vi "Get3DProfile.vi"(9 "dy":dbl, 10 "Origin":cluster{"X":sgl, "Y":sgl, "Z":sgl}, 11 "remaining elements":cluster{"x(mm)":dbl, "y(mm)":dbl, "z(mm)":dbl}[](array[cluster])) -> (0 "Z":dbl[](array[numeric]), 1 "Y":dbl[](array[numeric]), 2 "X":dbl[](array[numeric]), 3 "3D Profile":cluster{"x(mm)":dbl, "y(mm)":dbl, "z(mm)":dbl}[](array[cluster]))   [LabVIEW 2024]
panel:
  out "Z":dbl[](graph)
  out "Y":dbl[](graph)
  out "X":dbl[](graph)
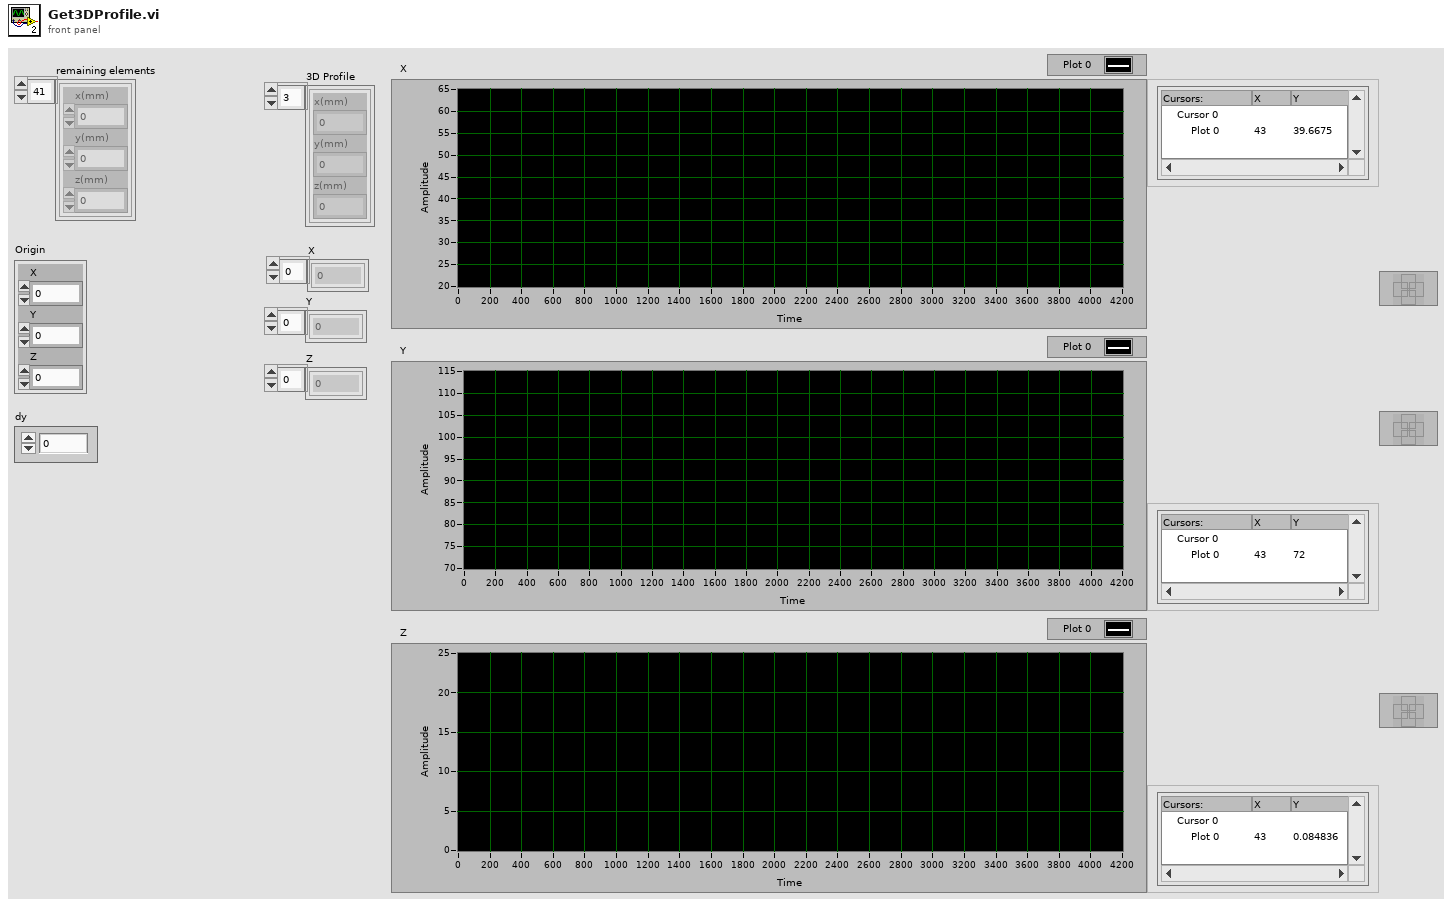
[diagram p1: front panel]
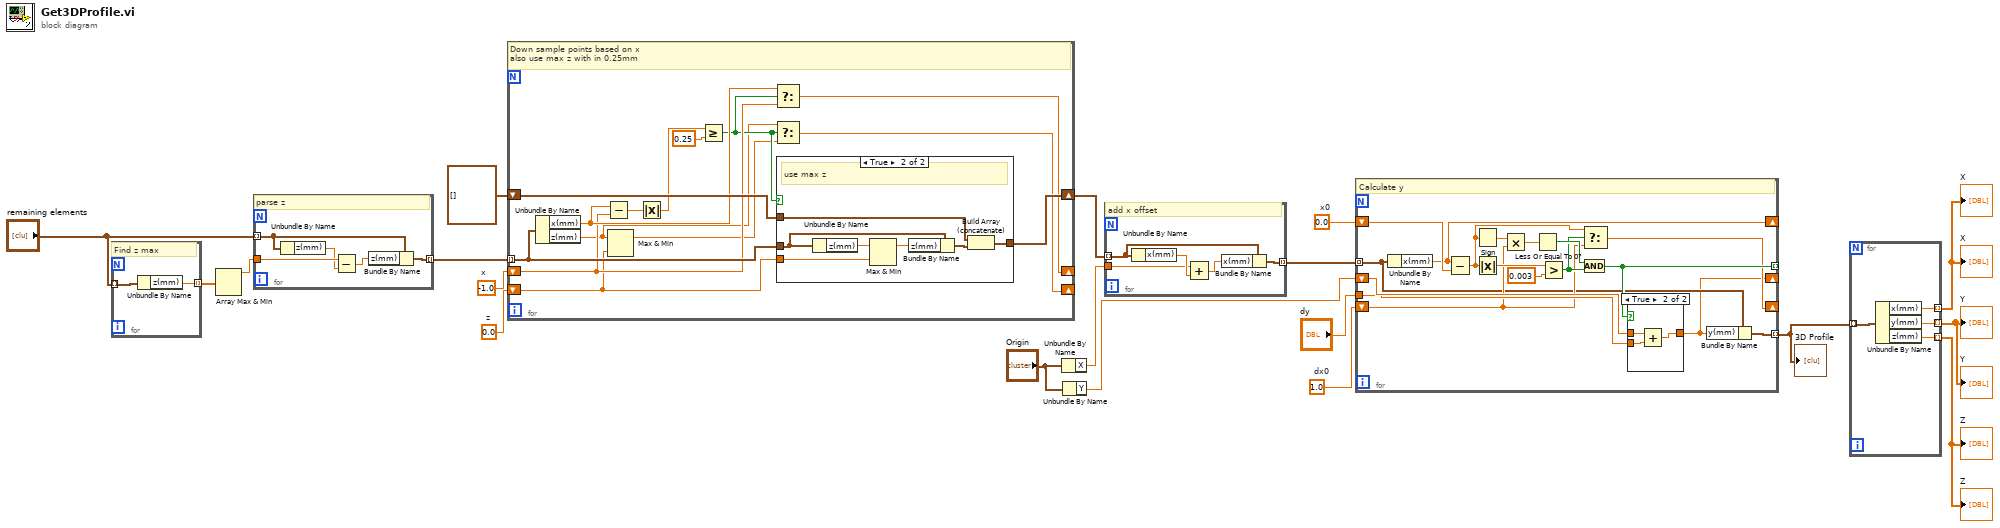
[diagram p0: block diagram]
diagram:
  w6 = 0.0  # z
  w16 = 1.0  # dx0
  w17 = 0.0  # x0
  w18 = -1.0  # x
  n1 = for {
    tunnel: "remaining elements" -> [w21] mode=indexing
    tunnel: [w20] -> w5 mode=indexing
    # "Find z max"
    n2 = Unbundle By Name(w21) -> ("z(mm)"=w20:dbl)
  }
  n3 = Array Max & Min(array=w5) -> (max value=w9:dbl)  [unwired: 3 out]
  n4 = for {
    tunnel: w9 -> [w26]
    tunnel: "remaining elements" -> [w24] mode=indexing
    tunnel: [w22] -> w7 mode=indexing
    # "parse z"
    n5 = Unbundle By Name(w24) -> ("z(mm)"=w25:dbl)
    n6 = Subtract(x=w26, y=w25) -> (x-y=w23:dbl)
    n7 = Bundle By Name(cluster=w24, "z(mm)"=w23) -> (w22:cluster{"x(mm)":dbl, "y(mm)":dbl, "z(mm)":dbl})
  }
  n8 = for {
    tunnel: w7 -> [w37] mode=indexing
    shift-right: [w33] -> _
    shift-left: w18 -> [w34]
    shift-right: [w36] -> w11
    shift-left: cluster{"x(mm)":dbl, "y(mm)":dbl, "z(mm)":dbl}[] [] -> [w38]
    shift-right: [w30] -> _
    shift-left: w6 -> [w27]
    # "Down sample points based on x\nalso use max z with in 0.25mm"
    n9 = Unbundle By Name(w37) -> ("x(mm)"=w35:dbl, "z(mm)"=w29:dbl)
    n10 = Subtract(x=w35, y=w34) -> (x-y=w40:dbl)
    n11 = Max & Min(x=w29, y=w27) -> (max(x,y)=w28:dbl)  [unwired: 1 out]
    n12 = Absolute Value(x=w40) -> (abs(x)=w32:dbl)
    n13 = Greater Or Equal?(x=w32, y=0.25) -> (x >= y?=w31:bool)
    n14 = Select(t=w35, s=w31, f=w34) -> (s? t:f=w33:dbl)
    n15 = Select(t=w29, s=w31, f=w28) -> (s? t:f=w30:dbl)
    n16 = case shown="True" w31 {
      tunnel: w38 -> [w41 w48]
      tunnel: w37 -> [_ w44]
      tunnel: [w41 w47] -> w36
      tunnel: w27 -> [_ w45]
      frame False {
      }
      frame True {
        # "use max z"
        n17 = Unbundle By Name(w44) -> ("z(mm)"=w46:dbl)
        n18 = Max & Min(x=w46, y=w45) -> (max(x,y)=w43:dbl)  [unwired: 1 out]
        n19 = Bundle By Name(cluster=w44, "z(mm)"=w43) -> (w42:cluster{"x(mm)":dbl, "y(mm)":dbl, "z(mm)":dbl})
        n20 = Build Array (concatenate)(w48, w42) -> (w47:cluster{"x(mm)":dbl, "y(mm)":dbl, "z(mm)":dbl}[])
      }
    }
  }
  n21 = Unbundle By Name("Origin") -> ("X"=w12:sgl)
  n22 = Unbundle By Name("Origin") -> ("Y"=w14:sgl)
  n23 = for {
    tunnel: w11 -> [w51] mode=indexing
    tunnel: w12 -> [w52]
    tunnel: [w49] -> w10 mode=indexing
    # "add x offset"
    n24 = Unbundle By Name(w51) -> ("x(mm)"=w53:dbl)
    n25 = Add(x=w52, y=w53) -> (x+y=w50:dbl)
    n26 = Bundle By Name(cluster=w51, "x(mm)"=w50) -> (w49:cluster{"x(mm)":dbl, "y(mm)":dbl, "z(mm)":dbl})
  }
  n27 = for {
    tunnel: w10 -> [w57] mode=indexing
    shift-right: [w54] -> _
    shift-left: w17 -> [w70]
    shift-right: [w59] -> _
    shift-left: w16 -> [w58]
    shift-right: [w56] -> _
    shift-left: w14 -> [w68]
    tunnel: "dy" -> [w67]
    tunnel: [w55] -> w4 mode=indexing
    tunnel: [w62] -> _ mode=indexing
    # "Calculate y"
    n28 = Unbundle By Name(w57) -> ("x(mm)"=w54:dbl)
    n29 = Subtract(x=w54, y=w70) -> (x-y=w60:dbl)
    n30 = Sign(1:w60) -> (0:w66:dbl)
    n31 = Absolute Value(x=w60) -> (abs(x)=w65:dbl)
    n32 = Multiply(x=w66, y=w58) -> (x*y=w69:dbl)
    n33 = Less Or Equal To 0?(x=w69) -> (x <= 0?=w63:bool)
    n34 = Greater?(x=w65, y=0.003) -> (0:w61:bool)
    n35 = And(x=w63, y=w61) -> (x .and. y?=w62:bool)
    n36 = Select(t=w60, s=w61, f=w58) -> (s? t:f=w59:dbl)
    n37 = case shown="True" w62 {
      tunnel: w68 -> [w71 w73]
      tunnel: [w71 w74] -> w56
      tunnel: w67 -> [_ w72]
      frame False {
      }
      frame True {
        n38 = Add(x=w73, y=w72) -> (x+y=w74:dbl)
      }
    }
    n39 = Bundle By Name(cluster=w57, "y(mm)"=w56) -> (w55:cluster{"x(mm)":dbl, "y(mm)":dbl, "z(mm)":dbl})
  }
  "3D Profile" <- w4
  n40 = for {
    tunnel: w4 -> [w78] mode=indexing
    tunnel: [w77] -> w2 mode=indexing
    tunnel: [w76] -> w1 mode=indexing
    tunnel: [w75] -> w3 mode=indexing
    n41 = Unbundle By Name(w78) -> ("x(mm)"=w77:dbl, "y(mm)"=w76:dbl, "z(mm)"=w75:dbl)
  }
  "Y" <- w1
  "X" <- w2
  "X" <- w2
  "Y" <- w1
  "Z" <- w3
  "Z" <- w3
